vi "Get Dynamic Member VIs Recursively.vi"(8 "error in (no error)":errorcluster, 11 "Source Class":refnum<vi>) -> (0 "error out":errorcluster, 3 "Dynamic Member VIs":refnum<vi>[](array[refnum]))   [LabVIEW 2020, in "Mock Class Generator.lvclass"]
uses:
  Mock Class Generator.lvclass
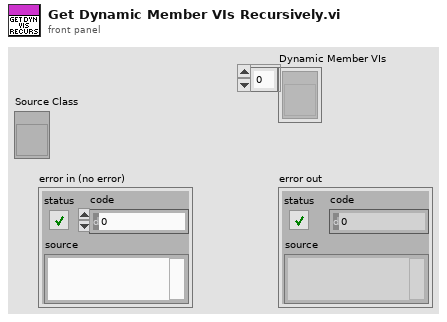
[diagram p1: front panel]
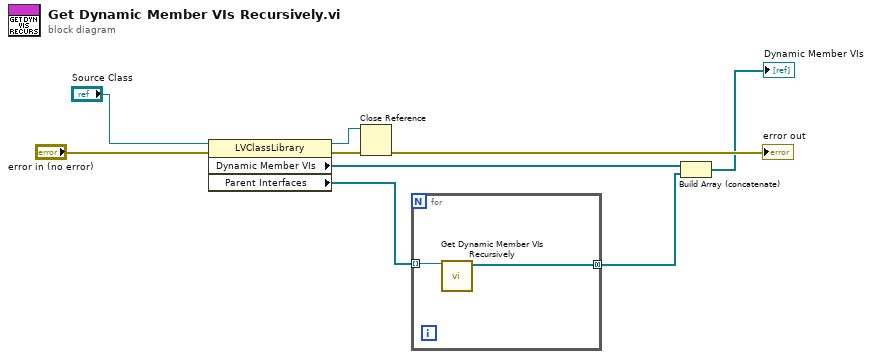
[diagram p0: block diagram]
diagram:
  n1 = property class="LVClassLibrary"(reference="Source Class", error in="error in (no error)") -> (reference out=w9:refnum<vi>, error out=w8:errorcluster, "Dynamic Member VIs"=w7:refnum<vi>[], "Parent Interfaces"=w5:refnum<vi>[])
  n2 = Close Reference(reference=w9, error in (no error)=w8) -> (error out=→"error out":errorcluster)
  n3 = for {
    tunnel: w5 -> [w11] mode=indexing
    tunnel: [w10] -> w1 mode=concatenating
    n4 = call "Get Dynamic Member VIs Recursively.vi"("Source Class"=w11) -> ("Dynamic Member VIs"=w10:refnum<vi>[])  [unwired: 9 in, 1 out]
  }
  n5 = Build Array (concatenate)(w7, w1) -> (→"Dynamic Member VIs":refnum<vi>[])
